vi "Start Sync.vi"(8 "error in (no error)":errorcluster, 11 "ServiceName Template in":refnum<class "ServiceName Template.lvclass">) -> (0 "error out":errorcluster, 3 "ServiceName Template out":refnum<class "ServiceName Template.lvclass">)   [LabVIEW 2024, in "ServiceName Template.lvclass"]
uses:
  ServiceName Template.lvclass
  ServiceName Template.lvclass/ServiceName Template.ctl
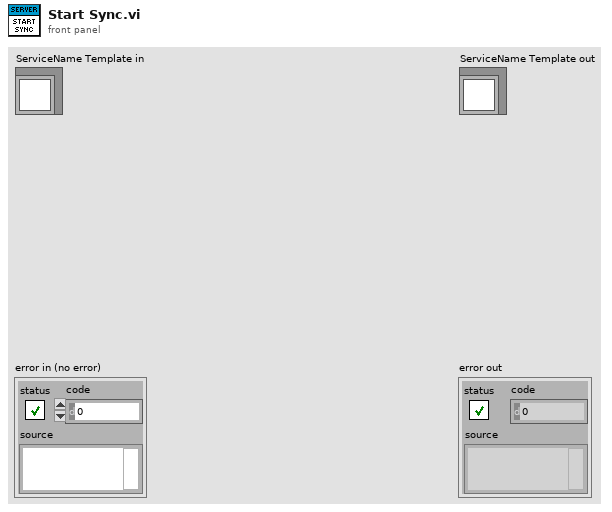
[diagram p1: front panel]
types:
  T1 = typedef "ServiceName Template.lvclass/Server Internal UEs.ctl" = cluster{"package_service_method Internal UE":refnum<user-event>}
  T2 = typedef "ServiceName Template.lvclass/Server gRPC UEs.ctl" = cluster{"package_service_method":refnum<user-event>}
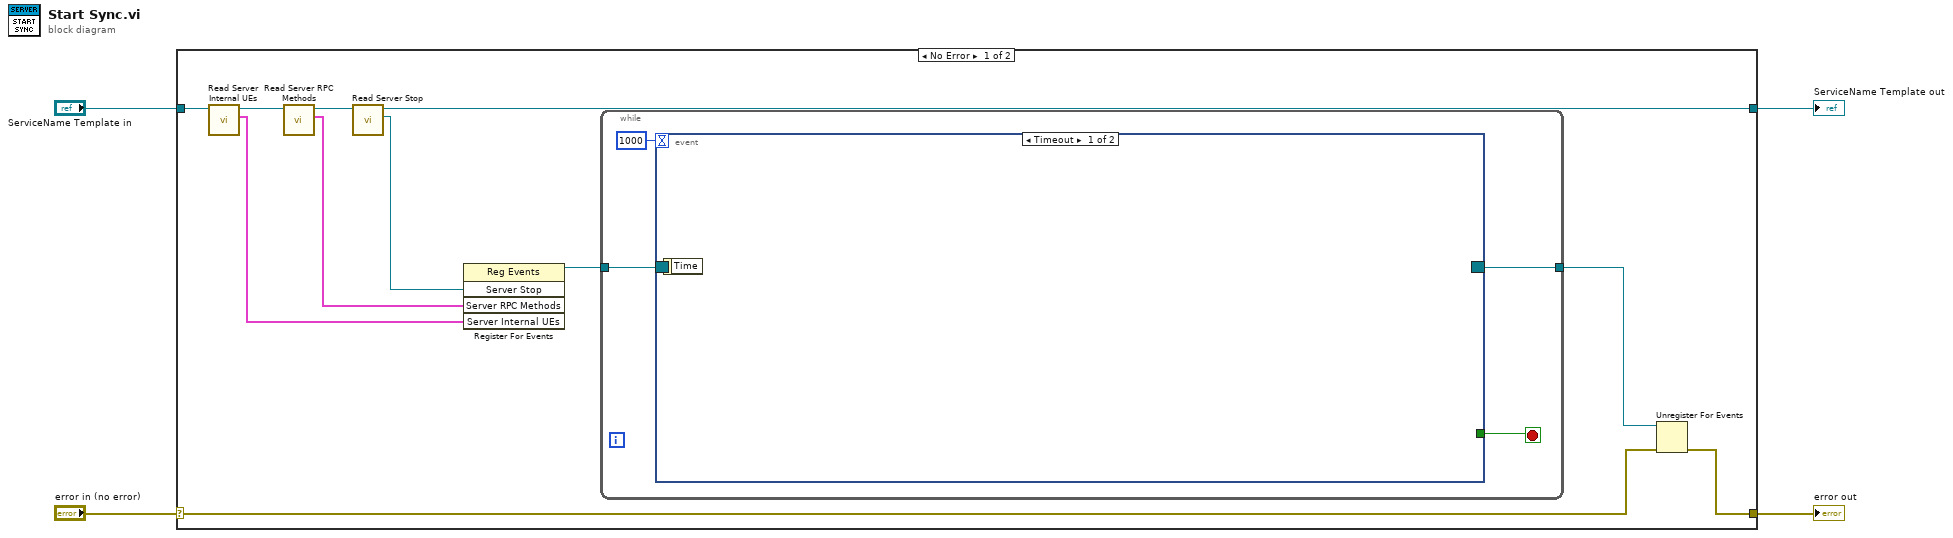
[diagram p0: block diagram]
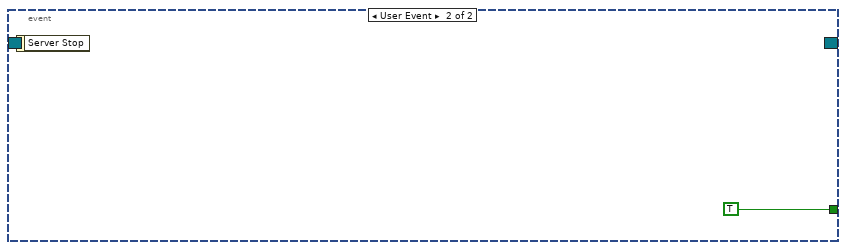
[diagram p2: hidden frame]
diagram:
  n1 = case shown="No Error" "error in (no error)" {
    selector: "error in (no error)" -> [w9 w22]
    tunnel: [w8 w22] -> w3
    tunnel: [w6 w21] -> w1
    tunnel: "ServiceName Template in" -> [w15 w21]
    frame No Error {
      n2 = call "Read Server Internal UEs.vi"("ServiceName Template in"=w15) -> ("Server Internal UEs"=w13:T1, "ServiceName Template out"=w14:refnum<class "ServiceName Template.lvclass">)  [unwired: 8 in, 1 out]
      n3 = call "Read Server RPC Methods.vi"("ServiceName Template in"=w14) -> ("Server RPC Methods"=w7:T2, "ServiceName Template out"=w12:refnum<class "ServiceName Template.lvclass">)  [unwired: 8 in, 1 out]
      n4 = call-dynamic "Read Server Stop.vi"("iService in"=w12) -> ("Server Stop"=w5:refnum<user-event>, "iService out"=w6:refnum<class "ServiceName Template.lvclass">)  [unwired: 8 in, 1 out]
      n5 = register-events(w5, w7, w13) -> (reference out=w11:refnum<event-registration>)  [unwired: 2 in, 1 out]
      n6 = while {
        tunnel: w11 -> [w19]
        tunnel: [w17] -> w10
        stop <- w18 stop-if-true
        n7 = event "RPC Methods Event Structure" shown="[0] Timeout" {
          selector: w19 -> [_ _]
          dyn-events: [_ _] -> w17
          timeout: 1000 -> [_ _]
          tunnel: [_ TRUE] -> w18
          event Timeout {
            n8 = event-data() -> ()  [unwired: 1 in, 1 out]
          }
          event User Event {
            n9 = event-data() -> ()  [unwired: 1 in, 1 out]
          }
        }
      }
      n10 = Unregister For Events(event registration refnum=w10, error in=w9) -> (error out=w8:errorcluster)
    }
    frame Error {
    }
  }
  "error out" <- w3
  "ServiceName Template out" <- w1
